vi "Magneto Encephalogram (MEG) Signal Analysis.vi"() -> ()   [LabVIEW 2023]
doc: "This example shows the applications of independent component analysis (ICA) in analyzing magneto encephalogram (MEG) signal analysis.\n\nMEG signals are the magnetic signals generated from electric dipoles around a human brain. These magnetic signals indicate activities in the brain. All cognitive activities in the human brain generate magnetic signals. Besides those cognitive activities, heartbeats, eye blinking, and breathing also generate magnetic signals. These signals are superimposed on the measured brain signal. To distinguish the brain signal from other signals, you can perform ICA on the MEG signals to remove the unwanted signals not originating in the brain activities. For example, you can remove the heartbeat signal from the MEG signals and perform further analysis on the residual signals. \n\nThe data used in this example has 148 channels from 148 sensors located in a helmet system, which takes the signal at the scalp. This example uses the TSA Independent Component Analysis VI to perform ICA on the MEG signals, removes the independent components corresponding to the heartbeat and breath, and reconstructs the MEG signals that correspond to the brain activities.\n\n<b>Instructions:</b>\n1) Run this VI.\n2) Observe the resulting independent components and the reconstructed MEG signals.\n3) Browse the Block Diagram of this example to learn how to remove some independent components and how to reconstruct signals."
uses:
  <vilib>/addons/Time Series Analysis/Utilities.llb/TSA Data.ctl
  <vilib>/Analysis/baseanly.llb/Real A x B.vi
  <vilib>/addons/Time Series Analysis/Statistical Analysis.llb/TSA Independent Component Analysis (Waveform).vi
  <vilib>/addons/_Advanced Signal Processing/NI_AdvSigProcTSA.lvlib
  <vilib>/Analysis/NI_AALBase.lvlib
panel:
  out "Removed Independent Components":waveform(dbl)[](graph)
  in  "IC to remove (index)":dbl[](array[numeric])=[0.0, 1.0, 8.0, 15.0]
  out "Reconstructed MEG Signals":waveform(dbl)[](graph)
  in  "Number of IC to search":i32=20
  out "Original MEG Signals":waveform(dbl)[](graph)
  out "Independent Components (IC)":waveform(dbl)[](graph)
  # "Overview: Shows the applications of independent component analysis (ICA) in analyzing magneto encephalogram (MEG) signal analysis.\nRequirements: LabVIEW Full Development System, Advanced Signal Processing Toolkit\nInstructions: \n1. Run this VI.\n2. Observe the resulting independent components and the reconstructed MEG signals.\n3. Browse the block diagram of this example to learn how to remove some independent components and how to reconstruct signals."
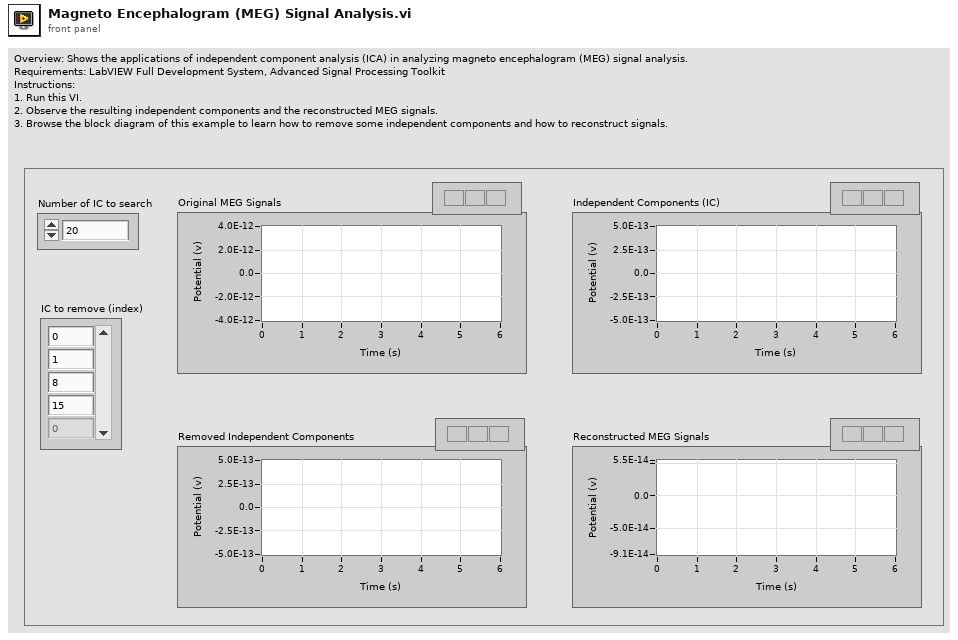
[diagram p1: front panel]
types:
  T1 = typedef "NI_AdvSigProcTSA.lvlib/TSA Data.ctl" = u16
  T2 = typedef "NI_Matrix.lvlib/RealMatrix.ctl" = dbl[][]
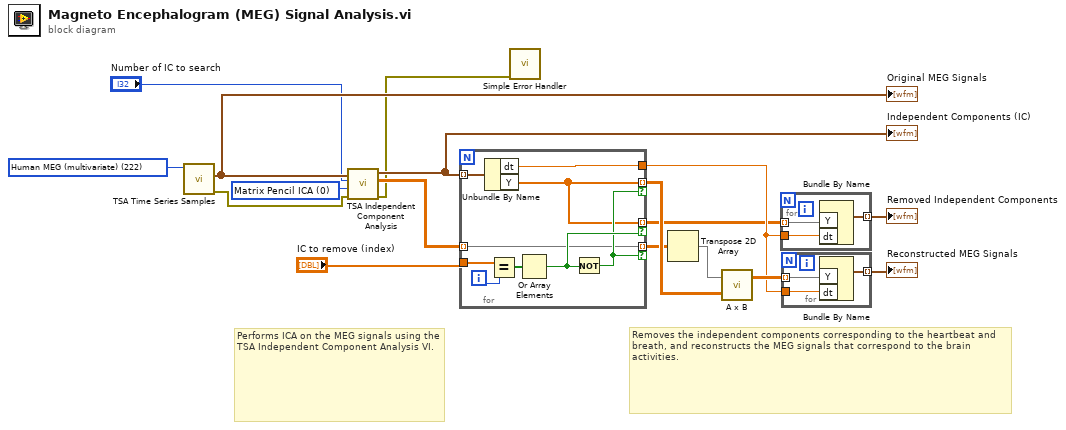
[diagram p0: block diagram]
diagram:
  w7 = T1 222 items=["Kobe Earthquake"=201, "EEG"=210, "Bearing Vibration (simulated)"=211, "Period Product Sales"=214, "Beam Vibration (nonlinear)"=217, "Beam Vibration (linear)"=218, "Signal With Echo"=219, "Engine Knocking"=220, "Power Line"=221, "-"=200, "Beam Deflections (multivariate)"=207, "Structure Vibration (multivariate)"=208, "Human MEG (multivariate)"=222] ("data")
  w17 = u16 0 items=["Matrix Pencil ICA", "Fast ICA"] ("method")
  # "Removes the independent components corresponding to the heartbeat and breath, and reconstructs the MEG signals that correspond to the brain activities."
  # "Performs ICA on the MEG signals using the TSA Independent Component Analysis VI."
  n1 = call <vilib>:"TSA Time Series Samples.vi"("data"=w7) -> ("error out"=w5:errorcluster, "multivariate time series"=w16:waveform(dbl)[])  [unwired: 1 in, 8 out]
  "Original MEG Signals" <- w16
  n2 = call-poly <vilib>:"TSA Independent Component Analysis.vi"("error in (no error)"=w5, "ICA method"=w17, "number of IC"="Number of IC to search", "Xt"=w16) -> ("error out"=w6:errorcluster, "separating matrix"=w13:dbl[][], "Xt out"=w12:waveform(dbl)[])  [unwired: 5 out]
  "Independent Components (IC)" <- w12
  n3 = for {
    tunnel: w12 -> [w25] mode=indexing
    tunnel: "IC to remove (index)" -> [w24]
    tunnel: w13 -> [w19] mode=indexing
    tunnel: [w22] -> w8
    tunnel: [w18] -> w4 mode=indexing if=w20
    tunnel: [w18] -> w3 mode=indexing if=w21
    tunnel: [w19] -> w2 mode=indexing if=w20
    i -> [w23]
    n4 = Unbundle By Name(w25) -> ("dt"=w22:dbl, "Y"=w18:dbl[])
    n5 = Equal?(x=w24, y=w23) -> (x = y?=w26:bool[])
    n6 = Or Array Elements(Boolean array=w26) -> (logical OR=w21:bool)
    n7 = Not(x=w21) -> (.not. x?=w20:bool)
  }
  n8 = call <vilib>:"Simple Error Handler.vi"("error in (no error)"=w6) -> ()  [unwired: 4 in, 5 out]
  n9 = Transpose 2D Array(2D array=w2) -> (transposed array=w1:dbl[][])
  n10 = call-poly <vilib>:"A x B.vi"("B"=w4, "A"=w1) -> ("A x B"=w11:T2)  [unwired: 1 out]
  n11 = for {
    tunnel: w3 -> [w29] mode=indexing
    tunnel: [w28] -> w9 mode=indexing
    tunnel: w8 -> [w27]
    n12 = Bundle By Name("Y"=w29, "dt"=w27) -> (w28:waveform(dbl))  [unwired: 1 out]
  }
  "Removed Independent Components" <- w9
  n13 = for {
    tunnel: w11 -> [w32] mode=indexing
    tunnel: [w31] -> w10 mode=indexing
    tunnel: w8 -> [w30]
    n14 = Bundle By Name("Y"=w32, "dt"=w30) -> (w31:waveform(dbl))  [unwired: 1 out]
  }
  "Reconstructed MEG Signals" <- w10
